vi "Apply.vi"(8 "error in":errorcluster, 11 "IMAQdx Triggered Continuous Acquisition in":refnum<class "IMAQdx Triggered Continuous Acquisition.lvclass">) -> (0 "error out":errorcluster, 3 "IMAQdx Triggered Continuous Acquisition out":refnum<class "IMAQdx Triggered Continuous Acquisition.lvclass">)   [LabVIEW 2025]
uses:
  IMAQdx Triggered Continuous Acquisition.lvclass
  Base/IMAQdx Base Configure Strategy.lvclass
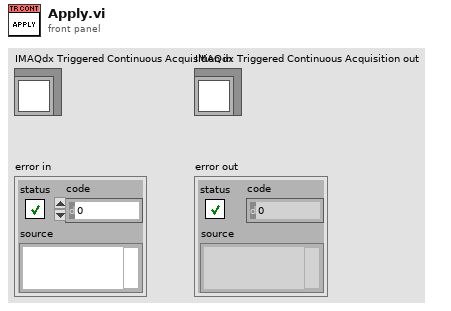
[diagram p1: front panel]
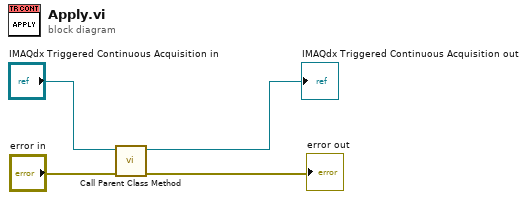
[diagram p0: block diagram]
diagram:
  n1 = call-parent "Call Parent Class Method"("error in"="error in", "IMAQdx Base Configure Strategy in"="IMAQdx Triggered Continuous Acquisition in") -> ("error out"=→"error out":errorcluster, "IMAQdx Base Configure Strategy out"=→"IMAQdx Triggered Continuous Acquisition out":refnum<class "IMAQdx Triggered Continuous Acquisition.lvclass">)  [unwired: 8 in]
